vi "DriveAxis.vi"(3 "Theta":dbl, 4 "Y":dbl, 5 "X":dbl) -> (0 "B":dbl, 1 "R":dbl, 2 "L":dbl)   [LabVIEW 2020]
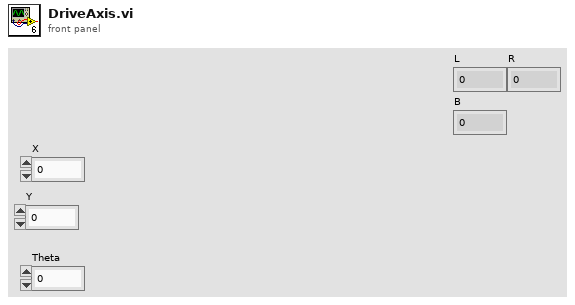
[diagram p1: front panel]
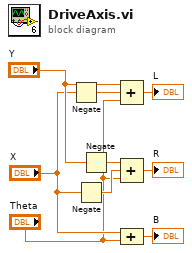
[diagram p0: block diagram]
diagram:
  n1 = Negate(x="X") -> (-x=w6:dbl)
  n2 = Negate(x="X") -> (-x=w5:dbl)
  n3 = Negate(x="Y") -> (-x=w8:dbl)
  n4 = Compound Arithmetic op=ADD("Y", w6, "Theta") -> (→"L":dbl)
  n5 = Compound Arithmetic op=ADD(w8, w5, "Theta") -> (→"R":dbl)
  n6 = Compound Arithmetic op=ADD("X", "Theta") -> (→"B":dbl)
